vi "CONCATENAR NUMEROS.vi"(8 "Enum":enum8{"APAGADO", "ENCENDIDO"}(ring), 11 "Numeric":u8) -> (1 "number":u8)   [LabVIEW 2019]
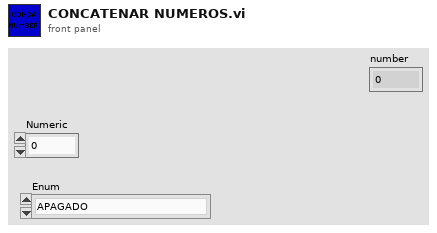
[diagram p1: front panel]
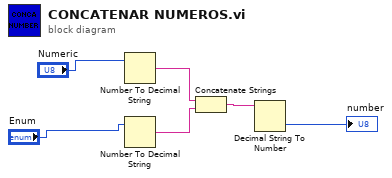
[diagram p0: block diagram]
diagram:
  n1 = Number To Decimal String(number="Numeric") -> (decimal integer string=w5:string)  [unwired: 1 in]
  n2 = Number To Decimal String(number="Enum") -> (decimal integer string=w4:string)  [unwired: 1 in]
  n3 = Concatenate Strings(w5, w4) -> (w3:string)
  n4 = Decimal String To Number(string=w3) -> (number=→"number":i32)  [unwired: 2 in, 1 out]
